vi "SCC File Status.vi"(8 "error in (no error)":errorcluster, 10 "files":path[](array[path]), 11 "source control reference in":T2) -> (0 "error out":errorcluster, 1 "file status":T1[](array[typedef]), 2 "status message":string, 3 "source control reference out":T2, 4 "files status flags":i32[](array[numeric]))   [LabVIEW 2017, in "NI_SCC.lvlib"]
doc: "Returns the current source control status of specified files, including whether a file is in source control, whether it is checked out, and whether it is the latest version available in source control."
uses:
  <vilib>/SourceControl/sccapi/NI_SCC.lvlib
  <vilib>/SourceControl/sccapi/SCCAPI Refnum.ctl
  <vilib>/SourceControl/sccapi/SCCAPI SCC File Status.ctl
  <vilib>/SourceControl/sccapi/SCCAPI SCC Operations.ctl
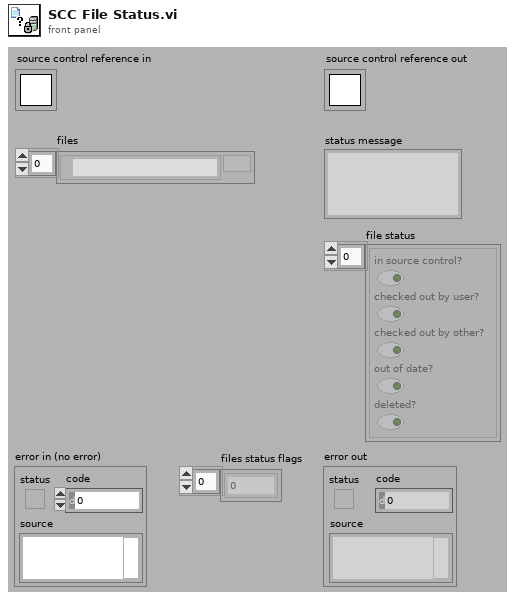
[diagram p1: front panel]
types:
  T1 = typedef "NI_SCC.lvlib/SCCAPI SCC File Status.ctl" = cluster{"in source control?":bool, "checked out by user?":bool, "checked out by other?":bool, "out of date?":bool, "deleted?":bool}
  T2 = typedef "NI_SCC.lvlib/SCCAPI Refnum.ctl" = refnum<k1>
  T3 = typedef "NI_SCC.lvlib/SCCAPI SCC Operations.ctl" = enum16{"Add", "Check In", "Check Out", "Close Project", "Compare Files", "Compare VIs", "Configure Project", "File History", "File Properties", "File Status", "Find All Providers", "Get Advanced Command Options", "Get File Copy", "Get Latest Version", "Get Project Name", "Get StaticVI Path", "Initialize", "Not A Source Control Reference", "Open Project", "Provider Supports Functionality", "Remove", "Run Provider", "Undo Check Out", "Uninitialize", "Is File In Local Path"}
  T4 = typedef "SCCAPI SCC File Status.ctl" = cluster{"source controlled":bool, "checked out by user":bool, "checked out by other":bool, "out of date":bool, "deleted":bool}
  T5 = typedef "SCCAPI Refnum.ctl" = refnum<k1>
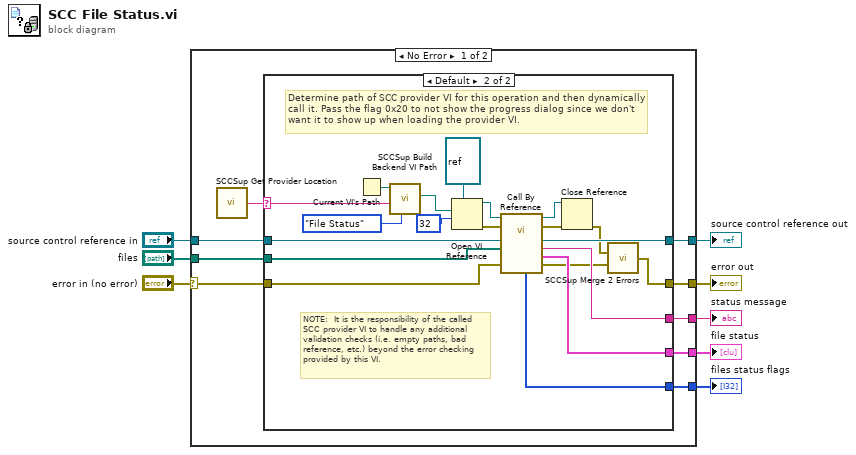
[diagram p0: block diagram]
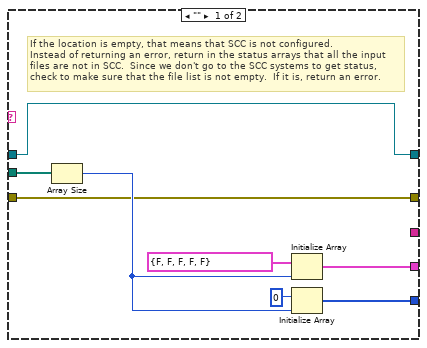
[diagram p2: hidden frame]
diagram:
  n1 = case shown="No Error" "error in (no error)" {
    selector: "error in (no error)" -> [w10 w47]
    tunnel: [w17 w47] -> w7
    tunnel: "source control reference in" -> [w16 w46]
    tunnel: [w15 _] -> w5
    tunnel: [w14 w46] -> w4
    tunnel: "files" -> [w13 _]
    tunnel: [w12 _] -> w2
    tunnel: [w9 _] -> w1
    frame No Error {
      n2 = call <vilib>:"SCCSup Get Provider Location.vi"() -> ("provider location"=w11:string)  [unwired: 6 in]
      n3 = case shown="Default" w11 {
        selector: w11 -> [_ w29]
        tunnel: [w23 w45] -> w17
        tunnel: w16 -> [w24 w37]
        tunnel: [_ w44] -> w15
        tunnel: [w24 w38] -> w14
        tunnel: w13 -> [w22 w36]
        tunnel: [w20 w35] -> w12
        tunnel: w10 -> [w23 w28]
        tunnel: [w21 w27] -> w9
        frame "" {
          # "If the location is empty, that means that SCC is not configured.  \nInstead of returning an error, return in the status arrays that all the input files are not in SCC.  Since we don't go to the SCC systems to get status, check to make sure that the file list is not empty.  If it is, return an error."
          n4 = Array Size(array=w22) -> (size(s)=w25:i32)
          n5 = Initialize Array(T1 {"in source control?"=FALSE, "checked out by user?"=FALSE, "checked out by other?"=FALSE, "out of date?"=FALSE, "deleted?"=FALSE} ("file status TD"), w25) -> (w20:T1[])
          n6 = Initialize Array(0, w25) -> (w21:i32[])
        }
        frame Default {
          # "NOTE:  It is the responsibility of the called SCC provider VI to handle any additional validation checks (i.e. empty paths, bad reference, etc.) beyond the error checking provided by this VI."
          # "Determine path of SCC provider VI for this operation and then dynamically call it. Pass the flag 0x20 to not show the progress dialog since we don't want it to show up when loading the provider VI."
          n7 = Current VI's Path() -> (path=w30:path)
          n8 = call <vilib>:"SCCSup Build Backend VI Path.vi"("scc operation"=SCCAPI_SCC_Operations."File Status", "provider location"=w29, "caller path"=w30) -> ("scc backend VI path"=w32:path)  [unwired: 8 in]
          n9 = Open VI Reference(type specifier VI Refnum (for type only)=refnum<vi> refnum, vi path=w32, options=32) -> (vi reference=w42:refnum<vi>, error out=w41:errorcluster)  [unwired: 3 in]
          n10 = call-by-ref "?"(reference=w42, error in=w41, "error in (no error)"=w28, "files"=w36, "source control reference in"=w37) -> (reference out=w40:refnum<vi>, error out=w39:errorcluster, 0:"error out"=w33:errorcluster, "file status"=w35:T4[], "status message"=w44:string, "source control reference out"=w38:T5, "files status flags"=w27:i32[])  [unwired: 4 in]
          n11 = Close Reference(reference=w40, error in (no error)=w39) -> (error out=w34:errorcluster)
          n12 = call <vilib>:"SCCSup Merge 2 Errors.vi"("Error IO 1"=w34, "Error IO 2"=w33) -> ("Error IO out"=w45:errorcluster)  [unwired: 13 in]
        }
      }
    }
    frame Error {
    }
  }
  "error out" <- w7
  "status message" <- w5
  "source control reference out" <- w4
  "file status" <- w2
  "files status flags" <- w1
